vi "tlc_Error Module.vi"(7 "Command (Handle Errors)":T4=enum."Handle Errors", 8 "error in (no error)":errorcluster, 9 "tlc_Consumer Queue Reference.ctl":T2, 10 "tlc_Display Queue Reference.ctl":T1, 11 "tlc_User Event Reference.ctl":T3) -> (0 "error out":errorcluster, 2 "status":bool)   [LabVIEW 2010]
doc: "If an error occurs, this module will gracefully shut down the TLC application by stopping the producer, consumer, and display loops."
uses:
  tlc_Error Module Command Control.ctl
  Controls/tlc_User Event Reference.ctl
  Controls/tlc_Consumer Queue Reference.ctl
  Controls/tlc_Consumer Control.ctl
  Application Command/Application Command.lvclass
  Controls/tlc_Display Queue Reference.ctl
  Controls/tlc_User Interface Command.ctl
  Controls/tlc_User Interface Data Type.ctl
  Exit/Exit App.lvclass
  Stop/Stop.lvclass
panel:
  # "Output"
  # "Input"
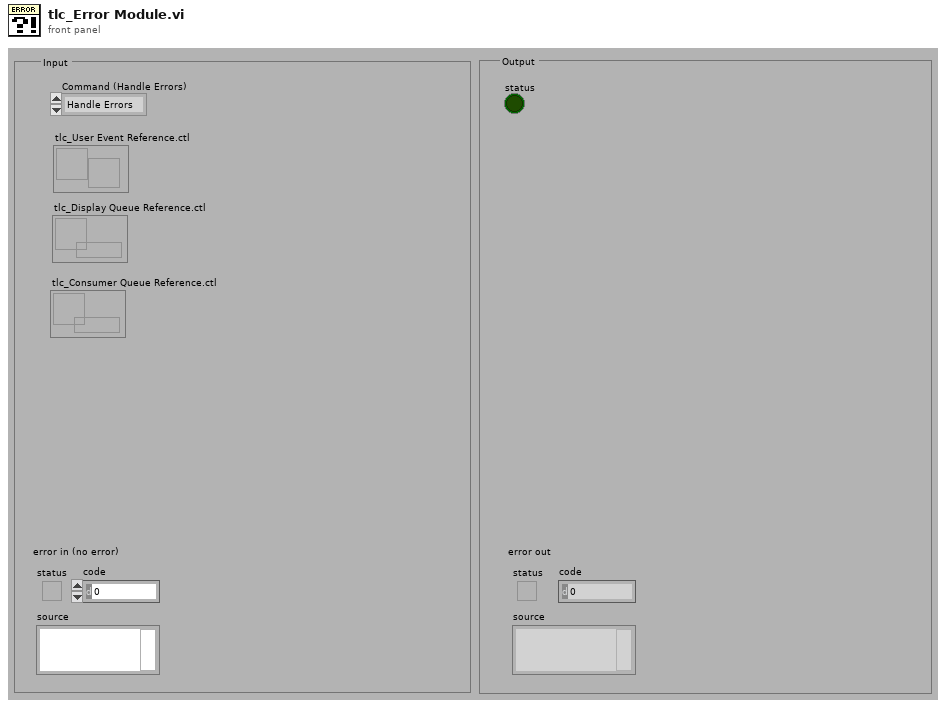
[diagram p1: front panel]
types:
  T1 = typedef "tlc_Display Queue Reference.ctl" = refnum<queue>
  T2 = typedef "tlc_Consumer Queue Reference.ctl" = refnum<queue>
  T3 = typedef "tlc_User Event Reference.ctl" = refnum<user-event>
  T4 = typedef "tlc_Error Module Command Control.ctl" = enum16{"Initialize", "Handle Errors", "Report Errors"}
  T5 = typedef "tlc_User Interface Command.ctl" = cluster{"Data Type":T6, "Data":variant}
  T6 = typedef "tlc_User Interface Data Type.ctl" = enum16{"Initialize", "Initialize Front Panel", "Update Front Panel Channels", "Select Cue in Cue List", "Enable/Disable Front Panel Controls", "Update Cue List", "Stop"}
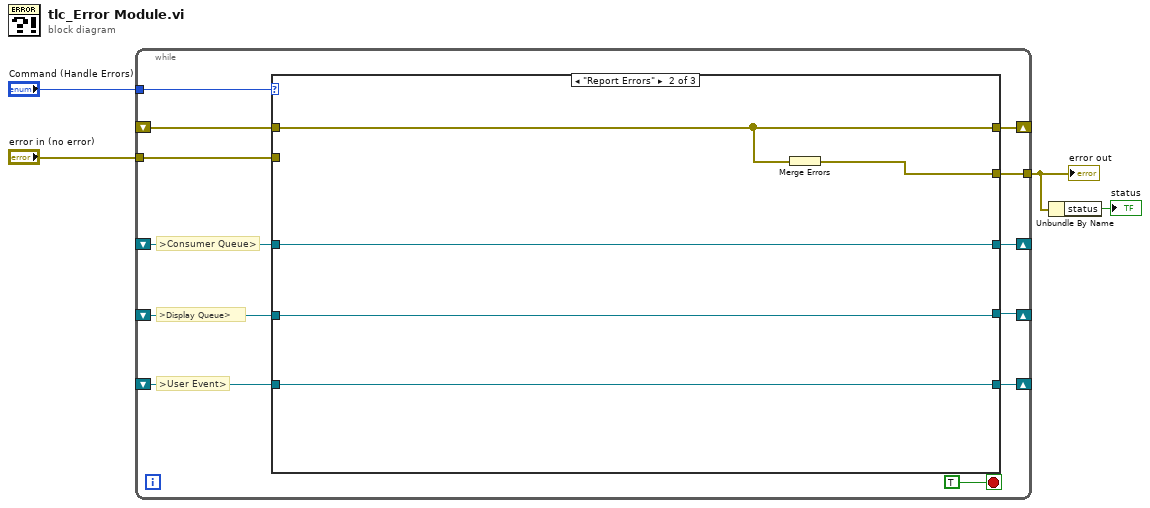
[diagram p0: block diagram]
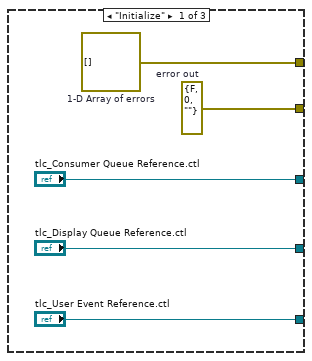
[diagram p2: hidden frame]
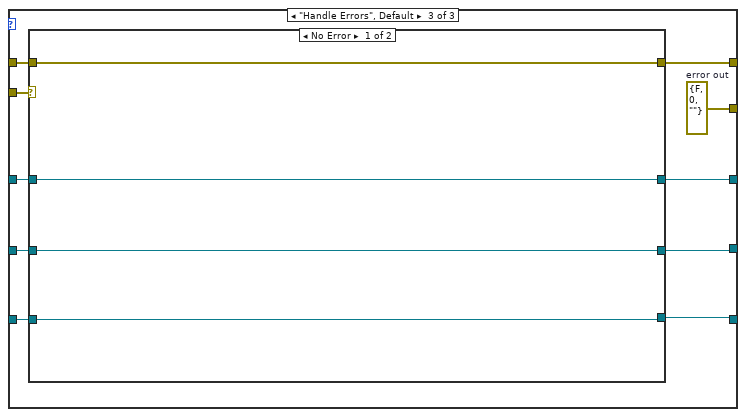
[diagram p3: hidden frame]
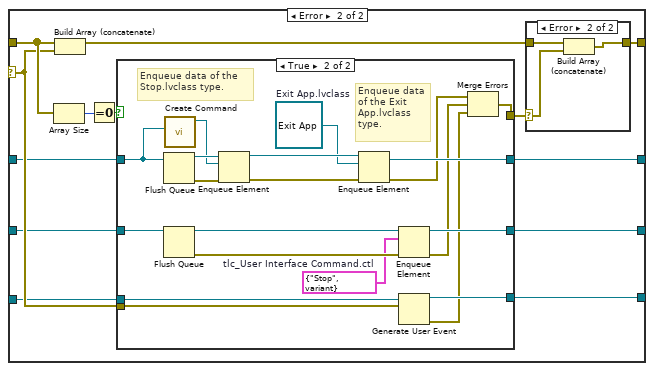
[diagram p4: hidden frame]
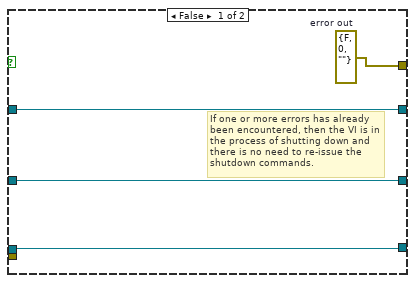
[diagram p6: hidden frame]
diagram:
  n1 = while {
    shift-right: [w12] -> _
    shift-left: _ -> [w14]
    tunnel: "error in (no error)" -> [w15]
    tunnel: "Command (Handle Errors)" -> [w13]
    tunnel: [w11] -> w2
    shift-right: [w10] -> _
    shift-left: _ -> [w7]
    shift-right: [w9] -> _
    shift-left: _ -> [w6]
    shift-right: [w8] -> _
    shift-left: _ -> [w5]
    stop <- TRUE stop-if-true
    # ">User Event>"
    # ">Display Queue>"
    # ">Consumer Queue>"
    n2 = case shown="\"Report Errors\"" w13 {
      tunnel: w15 -> [_ _ w36]
      tunnel: [w21 w25 w34] -> w12
      tunnel: w14 -> [_ w25 w35]
      tunnel: [w20 w26 w33] -> w11
      tunnel: ["tlc_Consumer Queue Reference.ctl" w24 w27] -> w10
      tunnel: ["tlc_Display Queue Reference.ctl" w23 w28] -> w9
      tunnel: ["tlc_User Event Reference.ctl" w22 w29] -> w8
      tunnel: w7 -> [_ w24 w32]
      tunnel: w6 -> [_ w23 w31]
      tunnel: w5 -> [_ w22 w30]
      frame "Initialize" {
        w20 = errorcluster {"status"=FALSE, "code"=0, "source"=""}  # error out
        w21 = errorcluster[] []  # 1-D Array of errors
      }
      frame "Report Errors" {
        n3 = Merge Errors(w25) -> (w26:errorcluster)
      }
      frame "Handle Errors", Default {
        w33 = errorcluster {"status"=FALSE, "code"=0, "source"=""}  # error out
        n4 = case shown="No Error" w36 {
          selector: w36 -> [_ w47]
          tunnel: [w40 w49] -> w34
          tunnel: w35 -> [w40 w53]
          tunnel: w32 -> [w39 w46]
          tunnel: w31 -> [w38 w45]
          tunnel: w30 -> [w37 w44]
          tunnel: [w37 w43] -> w29
          tunnel: [w38 w42] -> w28
          tunnel: [w39 w41] -> w27
          frame No Error {
          }
          frame Error {
            n5 = Array Size(array=w53) -> (size(s)=w51:i32)
            n6 = Build Array (concatenate)(w53, w47) -> (w50:errorcluster[])
            n7 = Equal To 0?(x=w51) -> (x = 0?=w52:bool)
            n8 = case shown="True" w52 {
              tunnel: [w61 w72] -> w48
              tunnel: w47 -> [_ w77]
              tunnel: w46 -> [w60 w62]
              tunnel: w45 -> [w59 w81]
              tunnel: w44 -> [w58 w78]
              tunnel: [w58 w75] -> w43
              tunnel: [w59 w74] -> w42
              tunnel: [w60 w73] -> w41
              frame False {
                w61 = errorcluster {"status"=FALSE, "code"=0, "source"=""}  # error out
                # "If one or more errors has already \nbeen encountered, then the VI is in \nthe process of shutting down and \nthere is no need to re-issue the \nshutdown commands."
              }
              frame True {
                w64 = refnum<class "Exit App.lvclass"> refnum  # Exit App.lvclass
                w76 = T5 {"Data Type"=enum."Stop", "Data"=variant}  # tlc_User Interface Command.ctl
                # "Enqueue data of the Exit App.lvclass type."
                # "Enqueue data of the Stop.lvclass type."
                n9 = Flush Queue(queue=w62) -> (queue out=w68:T2, error out=w67:errorcluster)  [unwired: 1 in, 1 out]
                n10 = Flush Queue(queue=w81) -> (queue out=w80:T1, error out=w79:errorcluster)  [unwired: 1 in, 1 out]
                n11 = call "Create Command.vi"("Command Queue"=w62) -> ("Stop.lvclass"=w63:refnum<class "Stop.lvclass">)  [unwired: 10 in]
                n12 = Enqueue Element(queue=w68, element=w63, error in (no error)=w67) -> (queue out=w65:T2, error out=w66:errorcluster)  [unwired: 1 in, 1 out]
                n13 = Enqueue Element(queue=w65, element=w64, error in (no error)=w66) -> (queue out=w73:T2, error out=w71:errorcluster)  [unwired: 1 in, 1 out]
                n14 = Enqueue Element(queue=w80, element=w76, error in (no error)=w79) -> (queue out=w74:T1, error out=w70:errorcluster)  [unwired: 1 in, 1 out]
                n15 = Generate User Event(user event=w78, event data cluster=w77) -> (user event out=w75:T3, error out=w69:errorcluster)  [unwired: 1 in]
                n16 = Merge Errors(w71, w70, w69) -> (w72:errorcluster)
              }
            }
            n17 = case shown="Error" w48 {
              selector: w48 -> [_ w55]
              tunnel: w50 -> [w54 w57]
              tunnel: [w54 w56] -> w49
              frame No Error {
              }
              frame Error {
                n18 = Build Array (concatenate)(w57, w55) -> (w56:errorcluster[])
              }
            }
          }
        }
      }
    }
  }
  "error out" <- w2
  n19 = Unbundle By Name(w2) -> ("status"=→"status":bool)
